vi "ALLPROPS0_Test.vi"(8 "error in (no error)":errorcluster) -> (0 "error out":errorcluster, 3 "Passed?":bool)   [LabVIEW 2016]
panel:
  out "Inputs":T1
  in  "Fluid of interest":string="HELIUM.FLD"
  out "Outputs":T2 {"Output" format="%_10g"}
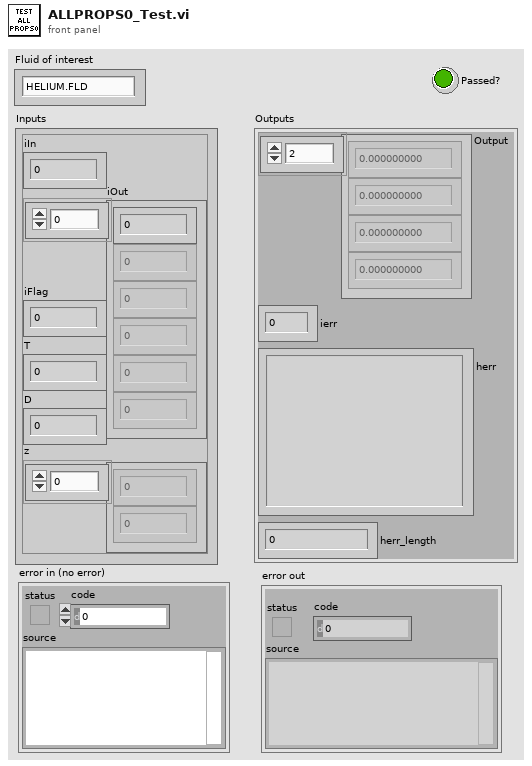
[diagram p1: front panel]
types:
  T1 = cluster{"iIn":i32, "iOut":i32[], "iFlag":i32, "T":dbl, "D":dbl, "z":dbl[]}
  T2 = cluster{"Output":dbl[], "ierr":i32, "herr":string, "herr_length":i32}
  T3 = cluster{"iEnum":i32, "ierr":i32, "herr":string, "hEnum_length":i32, "herr_length":i32}
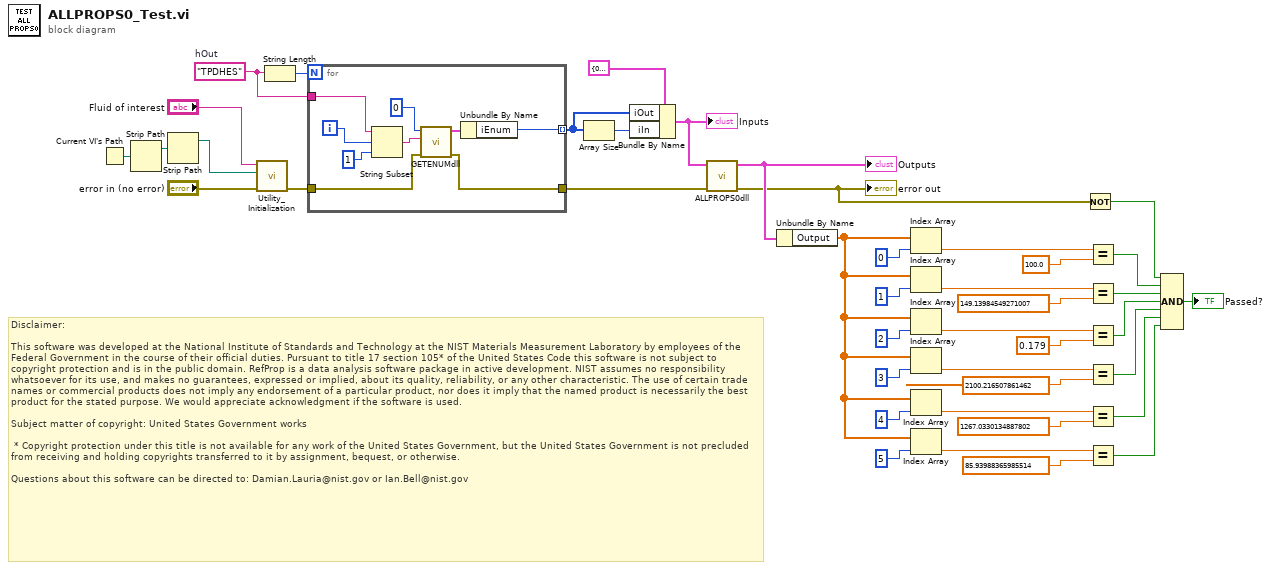
[diagram p0: block diagram]
diagram:
  w34 = "TPDHES"  # hOut
  # "Disclaimer:\n\nThis software was developed at the National Institute of Standards and Technology at the NIST Materials Measurement Laboratory by employees of the Federal Government in the course of their official duties. Pursuant to title 17 section 105* of the United States Code this software is not subject to copyright protection and is in the public domain. RefProp is a data analysis software package in active development. NIST assumes no responsibility whatsoever for its use, and makes no guarantees, expressed or implied, about its quality, reliability, or any other characteristic. The use of certain trade names or commercial products does not imply any endorsement of a particular product, nor does it imply that the named product is necessarily the best product for the stated purpose. We would appreciate acknowledgment if the software is used.\n \nSubject matter of copyright: United States Government works\n  \n * Copyright protection under this title is not available for any work of the United States Government, but the United States Government is not precluded from receiving and holding copyrights transferred to it by assignment, bequest, or otherwise.\n\nQuestions about this software can be directed to: Damian.Lauria@nist.gov or Ian.Bell@nist.gov"
  n1 = Current VI's Path() -> (path=w39:path)
  n2 = Strip Path(path=w39) -> (stripped path=w38:path)  [unwired: 1 out]
  n3 = Strip Path(path=w38) -> (stripped path=w37:path)  [unwired: 1 out]
  n4 = call "Utility_Initialization.vi"("error in (no error)"="error in (no error)", "path"=w37, "Fluidofinterest"="Fluid of interest") -> ("error out"=w35:errorcluster)  [unwired: 6 in, 2 out]
  n5 = String Length(string=w34) -> (length=w33:i32)
  n6 = for {
    N: w33 -> [_]
    tunnel: w34 -> [w51]
    tunnel: w35 -> [w50]
    tunnel: [w49] -> w41
    tunnel: [w48] -> w30 mode=indexing
    i -> [w43]
    n7 = String Subset(string=w51, offset (0)=w43, length (rest)=1 ("length (rest)")) -> (substring=w44:string)
    n8 = call "GETENUMdll.vi"("error in (no error)"=w50, "hEnum"=w44, "iFlag"=0) -> ("error out"=w49:errorcluster, "Outputs"=w45:T3)  [unwired: 7 in]
    n9 = Unbundle By Name(w45) -> ("iEnum"=w48:i32)
  }
  n10 = Array Size(array=w30) -> (size(s)=w32:i32)
  n11 = Bundle By Name(cluster=T1 {"iIn"=0, "iOut"=[0, 0, 0, 0, 0, 0, 0, 0, 0, 0, 0, 0, 0, 0, 0, 0, 0, 0, 0, 0, 0, 0, 0, 0, 0, 0, 0, 0, 0, 0, 0, 0, 0, 0, 0, 0, 0, 0, 0, 0, 0, 0, 0, 0, 0, 0, 0, 0, 0, 0, 0, 0, 0, 0, 0, 0, 0, 0, 0, 0, 0, 0, 0, 0, 0, 0, 0, 0, 0, 0, 0, 0, 0, 0, 0, 0, 0, 0, 0, 0, 0, 0, 0, 0, 0, 0, 0, 0, 0, 0, 0, 0, 0, 0, 0, 0, 0, 0, 0, 0, 0, 0, 0, 0, 0, 0, 0, 0, 0, 0, 0, 0, 0, 0, 0, 0, 0, 0, 0, 0, 0, 0, 0, 0, 0, 0, 0, 0, 0, 0, 0, 0, 0, 0, 0, 0, 0, 0, 0, 0, 0, 0, 0, 0, 0, 0, 0, 0, 0, 0, 0, 0, 0, 0, 0, 0, 0, 0, 0, 0, 0, 0, 0, 0, 0, 0, 0, 0, 0, 0, 0, 0, 0, 0, 0, 0, 0, 0, 0, 0, 0, 0, 0, 0, 0, 0, 0, 0, 0, 0, 0, 0, 0, 0, 0, 0, 0, 0, 0, 0], "iFlag"=0, "T"=100.0, "D"=0.179, "z"=[1.0, 0.0, 0.0, 0.0, 0.0, 0.0, 0.0, 0.0, 0.0, 0.0, 0.0, 0.0, 0.0, 0.0, 0.0, 0.0, 0.0, 0.0, 0.0, 0.0]} ("Inputs"), "iOut"=w30, "iIn"=w32) -> (w42:T1)
  "Inputs" <- w42
  n12 = call "ALLPROPS0dll.vi"("error in (no error)"=w41, "Inputs"=w42) -> ("error out"=w10:errorcluster, "Outputs"=w29:T2)  [unwired: 8 in]
  "Outputs" <- w29
  "error out" <- w10
  n13 = Unbundle By Name(w29) -> ("Output"=w22:dbl[])
  n14 = Index Array(array=w22, index=0) -> (element=w21:dbl)
  n15 = Index Array(array=w22, index=1) -> (element=w7:dbl)
  n16 = Index Array(array=w22, index=2) -> (element=w20:dbl)
  n17 = Index Array(array=w22, index=3) -> (element=w6:dbl)
  n18 = Index Array(array=w22, index=4) -> (element=w3:dbl)
  n19 = Index Array(array=w22, index=5) -> (element=w19:dbl)
  n20 = Not(x=w10) -> (.not. x?=w9:bool)
  n21 = Equal?(x=w21, y=100.0) -> (x = y?=w16:bool)
  n22 = Equal?(x=w7, y=149.13984549271007 ("element")) -> (x = y?=w15:bool)
  n23 = Equal?(x=w20, y=0.179) -> (x = y?=w14:bool)
  n24 = Equal?(x=w6, y=2100.216507861462 ("element 2")) -> (x = y?=w13:bool)
  n25 = Equal?(x=w3, y=1267.0330134887802 ("element 3")) -> (x = y?=w12:bool)
  n26 = Equal?(x=w19, y=85.93988365985514 ("element 4")) -> (x = y?=w11:bool)
  n27 = Compound Arithmetic op=AND(w9, w16, w15, w14, w13, w12, w11) -> (→"Passed?":bool)
